vi "rs3_make_faces.vi"(10 "Width":i32, 11 "Height":i32) -> (2 "all faces":i32[][](array[numeric]), 3 "Face Array":string[][](array[string]))   [LabVIEW 2017, in "libRealSense3.lvlib"]
uses:
  libRealSense3.lvlib
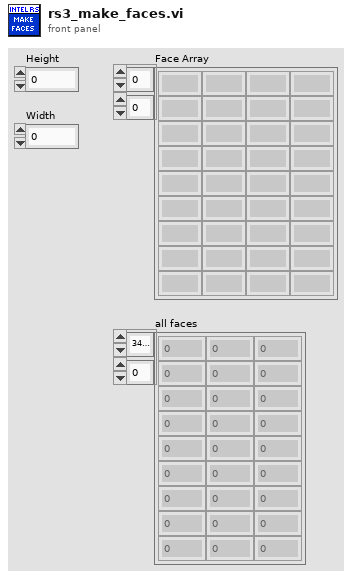
[diagram p1: front panel]
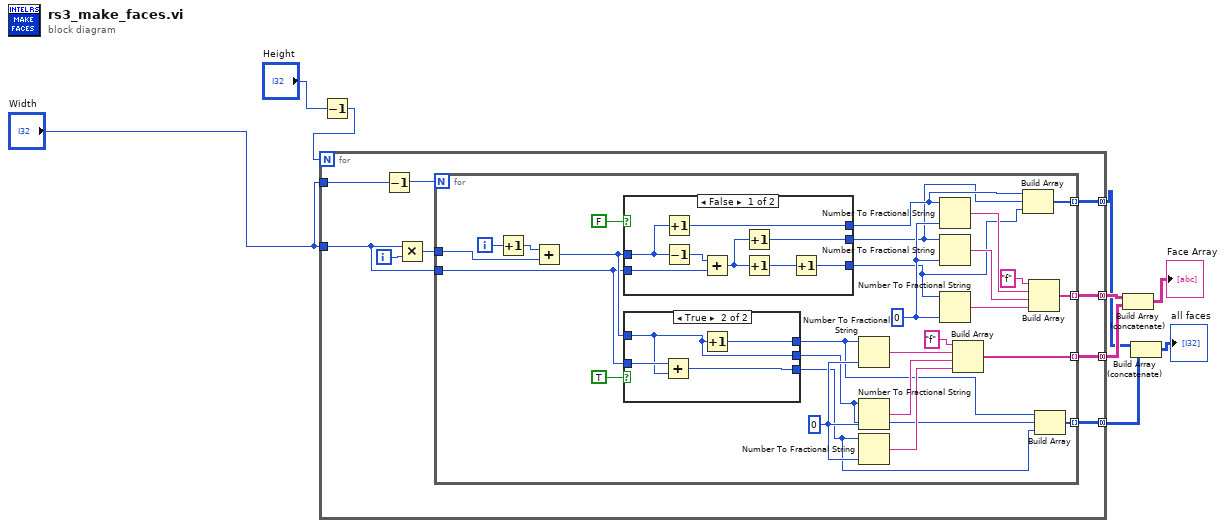
[diagram p0: block diagram]
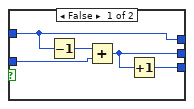
[diagram p2: hidden frame]
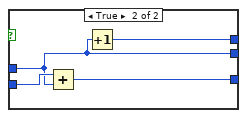
[diagram p3: hidden frame]
diagram:
  n1 = Decrement(x="Height") -> (x-1=w3:i32)
  n2 = for {
    N: w3 -> [_]
    tunnel: "Width" -> [w16]
    tunnel: "Width" -> [w18]
    tunnel: [w14] -> w6 mode=concatenating
    tunnel: [w13] -> w5 mode=concatenating
    tunnel: [w11] -> w2 mode=concatenating
    tunnel: [w10] -> w8 mode=concatenating
    i -> [w17]
    n3 = Decrement(x=w18) -> (x-1=w12:i32)
    n4 = Multiply(x=w16, y=w17) -> (x*y=w15:i32)
    n5 = for {
      N: w12 -> [_]
      tunnel: w16 -> [w36]
      tunnel: [w29] -> w14 mode=indexing
      tunnel: w15 -> [w40]
      tunnel: [w27] -> w13 mode=indexing
      tunnel: [w23] -> w11 mode=indexing
      tunnel: [w19] -> w10 mode=indexing
      i -> [w41]
      w28 = i16 0 ("precision (6)")
      w42 = i16 0 ("precision (6)")
      n6 = Increment(x=w41) -> (x+1=w39:i32)
      n7 = Add(x=w39, y=w40) -> (x+y=w37:i32)
      n8 = case shown="False" FALSE {
        tunnel: w36 -> [w62 w66]
        tunnel: [w55 w63] -> w25
        tunnel: [w59 w65] -> w26
        tunnel: w37 -> [w60 w63]
        tunnel: [w57 w64] -> w24
        frame False {
          n9 = Increment(x=w60) -> (x+1=w59:i32)
          n10 = Decrement(x=w60) -> (x-1=w61:i32)
          n11 = Add(x=w61, y=w62) -> (x+y=w56:i32)
          n12 = Increment(x=w56) -> (x+1=w55:i32)
          n13 = Increment(x=w56) -> (x+1=w58:i32)
          n14 = Increment(x=w58) -> (x+1=w57:i32)
        }
        frame True {
          n15 = Add(x=w66, y=w63) -> (x+y=w64:i32)
          n16 = Increment(x=w63) -> (x+1=w65:i32)
        }
      }
      n17 = case shown="True" TRUE {
        tunnel: w36 -> [w48 w54]
        tunnel: [w47 w51] -> w21
        tunnel: [w50 w53] -> w22
        tunnel: w37 -> [w50 w51]
        tunnel: [w46 w52] -> w20
        frame False {
          n18 = Decrement(x=w50) -> (x-1=w49:i32)
          n19 = Add(x=w49, y=w48) -> (x+y=w47:i32)
          n20 = Increment(x=w47) -> (x+1=w46:i32)
        }
        frame True {
          n21 = Add(x=w54, y=w51) -> (x+y=w52:i32)
          n22 = Increment(x=w51) -> (x+1=w53:i32)
        }
      }
      n23 = Number To Fractional String(number=w22, precision (6)=w28) -> (F-format string=w30:string)  [unwired: 2 in]
      n24 = Number To Fractional String(number=w21, precision (6)=w28) -> (F-format string=w31:string)  [unwired: 2 in]
      n25 = Number To Fractional String(number=w20, precision (6)=w28) -> (F-format string=w32:string)  [unwired: 2 in]
      n26 = Number To Fractional String(number=w26, precision (6)=w42) -> (F-format string=w45:string)  [unwired: 2 in]
      n27 = Number To Fractional String(number=w25, precision (6)=w42) -> (F-format string=w44:string)  [unwired: 2 in]
      n28 = Number To Fractional String(number=w24, precision (6)=w42) -> (F-format string=w43:string)  [unwired: 2 in]
      n29 = Build Array("f", w30, w31, w32) -> (w29:string[])
      n30 = Build Array(w26, w25, w24) -> (w23:i32[])
      n31 = Build Array("f", w45, w44, w43) -> (w27:string[])
      n32 = Build Array(w22, w21, w20) -> (w19:i32[])
    }
  }
  n33 = Build Array (concatenate)(w5, w6) -> (→"Face Array":string[][])
  n34 = Build Array (concatenate)(w2, w8) -> (→"all faces":i32[][])
